vi "Callback - Get Data by Name.vi"(8 "error in (no error)":errorcluster, 10 "Name":string, 11 "BluePlotHandle in":refnum<class "BluePlotHandle.lvclass">) -> (0 "error out":errorcluster, 2 "data history":T1, 3 "BluePlotHandle out":refnum<class "BluePlotHandle.lvclass">)   [LabVIEW 2021, in "BluePlot.lvlib" / "BluePlotHandle.lvclass"]
uses:
  BluePlotHandle.lvclass
  TypeDefs/plot datapoint.ctl
  BluePlot.lvlib
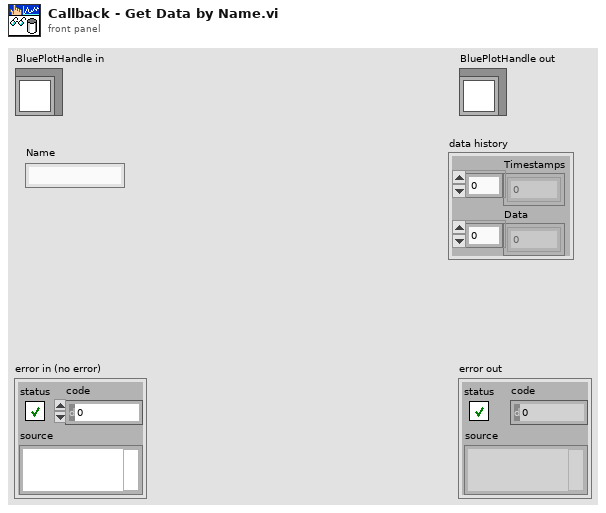
[diagram p1: front panel]
types:
  T1 = typedef "BluePlot.lvlib/plot datapoint.ctl" = cluster{"Timestamps":dbl[], "Data":dbl[]}
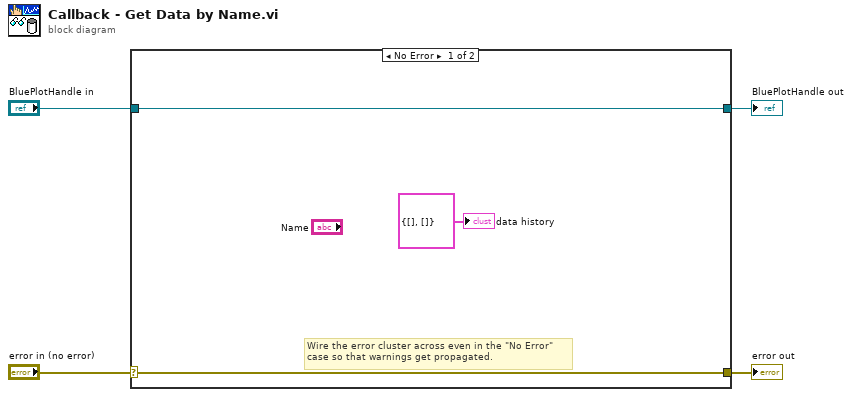
[diagram p0: block diagram]
diagram:
  n1 = case shown="No Error" "error in (no error)" {
    selector: "error in (no error)" -> [w6 w9]
    tunnel: [w6 w9] -> w3
    tunnel: [w7 w8] -> w1
    tunnel: "BluePlotHandle in" -> [w7 w8]
    frame No Error {
      # "Wire the error cluster across even in the \"No Error\"\ncase so that warnings get propagated."
      "data history" <- T1 {"Timestamps"=[], "Data"=[]} ("data history")
    }
    frame Error {
    }
  }
  "error out" <- w3
  "BluePlotHandle out" <- w1
